vi "get_all_qcm_status.vi"(8 "error in (no error)":errorcluster, 11 "VISA resource name":refnum<visa-resource-name>) -> (0 "error out":errorcluster, 2 "Status array":T1(array[cluster]), 3 "VISA resource name out":refnum<visa-resource-name>)   [LabVIEW 2018]
doc: "Query the status of all sensors."
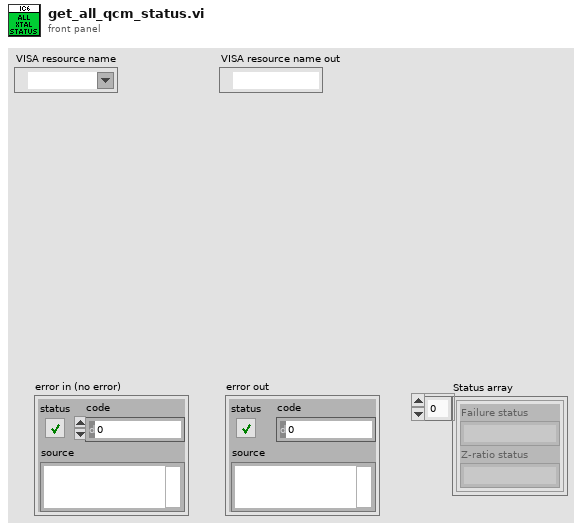
[diagram p1: front panel]
types:
  T1 = cluster{"Failure status":string, "Z-ratio status":string}[]
  T2 = enum16{"Source", "General", "Input name", "Process name", "Logic", "Material", "Material name", "Output name", "Process", "Sensor", "Output type", "User message", "Layer", ""}
  T3 = enum16{"Hello", "Query", "Remote action", "Status", "Update"}
  T4 = cluster{"Failure status":string, "Z-ratio status":string}
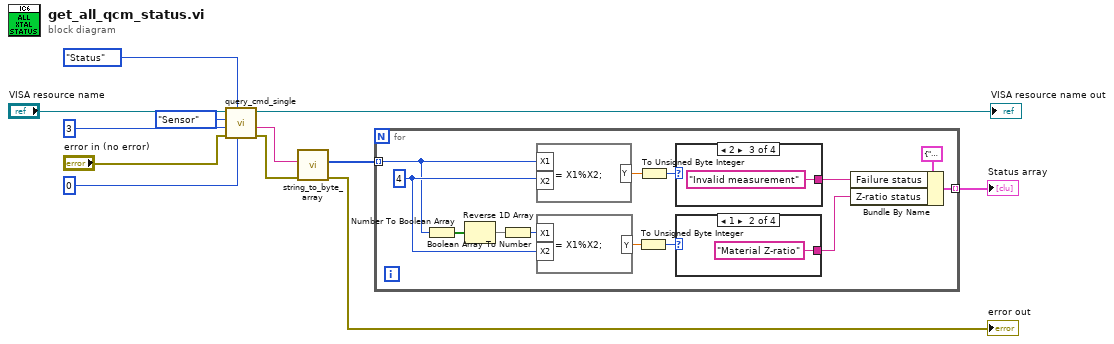
[diagram p0: block diagram]
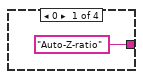
[diagram p2: hidden frame]
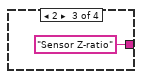
[diagram p3: hidden frame]
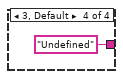
[diagram p4: hidden frame]
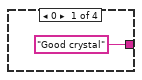
[diagram p5: hidden frame]
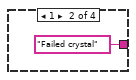
[diagram p6: hidden frame]
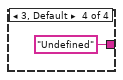
[diagram p7: hidden frame]
diagram:
  n1 = call "query_cmd_single.vi"("Parameter"=u8 0 ("Command ID"), "Command group"=T3."Status", "error in (no error)"="error in (no error)", "Command ID"=u8 3, "Command subgroup"=T2."Sensor", "VISA resource name"="VISA resource name") -> ("error out"=w6:errorcluster, "formatted response"=w1:string, "VISA resource name out"=→"VISA resource name out":refnum<visa-resource-name>)  [unwired: 1 in, 2 out]
  n2 = call "string_to_byte_array.vi"("error in (no error)"=w6, "Byte"=w1) -> ("error out"=→"error out":errorcluster, "Int array"=w2:u8[])  [unwired: 8 in]
  n3 = for {
    tunnel: w2 -> [w17] mode=indexing
    tunnel: [w13] -> w4 mode=indexing
    w18 = u8 4 ("input variable")
    n4 = Number To Boolean Array(number=w17) -> (Boolean array=w19:bool[])
    n5 = Reverse 1D Array(array=w19) -> (reversed array=w20:bool[])
    n6 = Boolean Array To Number(Boolean array=w20) -> (number=w21:u32)
    n7 = formula code="Y = X1%X2;"("X1"=w17, "X2"=w18) -> ("Y"=w23:dbl)
    n8 = formula code="Y = X1%X2;"("X1"=w21, "X2"=w18) -> ("Y"=w22:dbl)
    n9 = To Unsigned Byte Integer(number=w22) -> (unsigned 8bit integer=w25:u8)
    n10 = To Unsigned Byte Integer(number=w23) -> (unsigned 8bit integer=w24:u8)
    n11 = case shown="2" w24 {
      tunnel: ["Good crystal" ("String") "Failed crystal" ("String") "Invalid measurement" ("String") "Undefined" ("String")] -> w15
      frame 0 {
      }
      frame 1 {
      }
      frame 2 {
      }
      frame 3, Default {
      }
    }
    n12 = case shown="1" w25 {
      tunnel: ["Auto-Z-ratio" ("String") "Material Z-ratio" ("String") "Sensor Z-ratio" ("String") "Undefined" ("String")] -> w14
      frame 0 {
      }
      frame 1 {
      }
      frame 2 {
      }
      frame 3, Default {
      }
    }
    n13 = Bundle By Name(cluster=T4 {"Failure status"="", "Z-ratio status"=""}, "Failure status"=w15, "Z-ratio status"=w14) -> (w13:T4)
  }
  "Status array" <- w4
